vi "Evaluate Part 1.vi"() -> ()   [LabVIEW 2021]
uses:
  Proto/Group.lvclass
panel:
  out "sum":u64=21
  in  "String":string="???.### 1,1,3\n.??..??...?##. 1,1,3\n?#?#?#?#?#?#?#? 1,3,1,6\n????.#...#... 4,1,1\n????.######..#####. 1,6,5\n?###???????? 3,2,1"
  # "7408 too high"
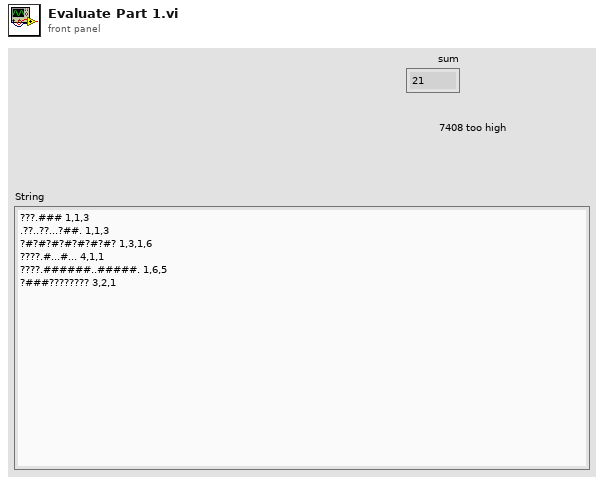
[diagram p1: front panel]
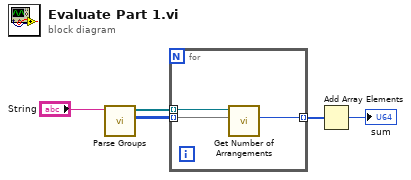
[diagram p0: block diagram]
diagram:
  n1 = call "Parse Groups.vi"("Input"="String") -> ("Counts"=w2:i64[][], "Groups"=w1:refnum<class "Group.lvclass">[])  [unwired: 9 in]
  n2 = for {
    tunnel: w1 -> [w8] mode=indexing
    tunnel: w2 -> [w7] mode=indexing
    tunnel: [w6] -> w4 mode=indexing
    n3 = call "Get Number of Arrangements.vi"("Group Sizes"=w7, "Proto in"=w8) -> ("Arrangements"=w6:u64)  [unwired: 7 in, 2 out]
  }
  n4 = Add Array Elements(numeric array=w4) -> (sum=→"sum":u64)
